vi "Get Spectrum.vi"(8 "error in (no error)":errorcluster, 11 "Micron Hyperion Driver in":refnum<class "Micron Hyperion Driver.lvclass">) -> (0 "error out":errorcluster, 2 "Spectrum Graph":cluster{dbl[], "Spectrum, db":dbl[]}[](graph), 3 "Micron Hyperion Driver out":refnum<class "Micron Hyperion Driver.lvclass">)   [LabVIEW 2016, in "Micron Hyperion Driver.lvclass"]
uses:
  Micron Hyperion Driver.lvclass
  Micron Hyperion Driver.lvclass/Micron Hyperion Driver.ctl
  Read Address.vi
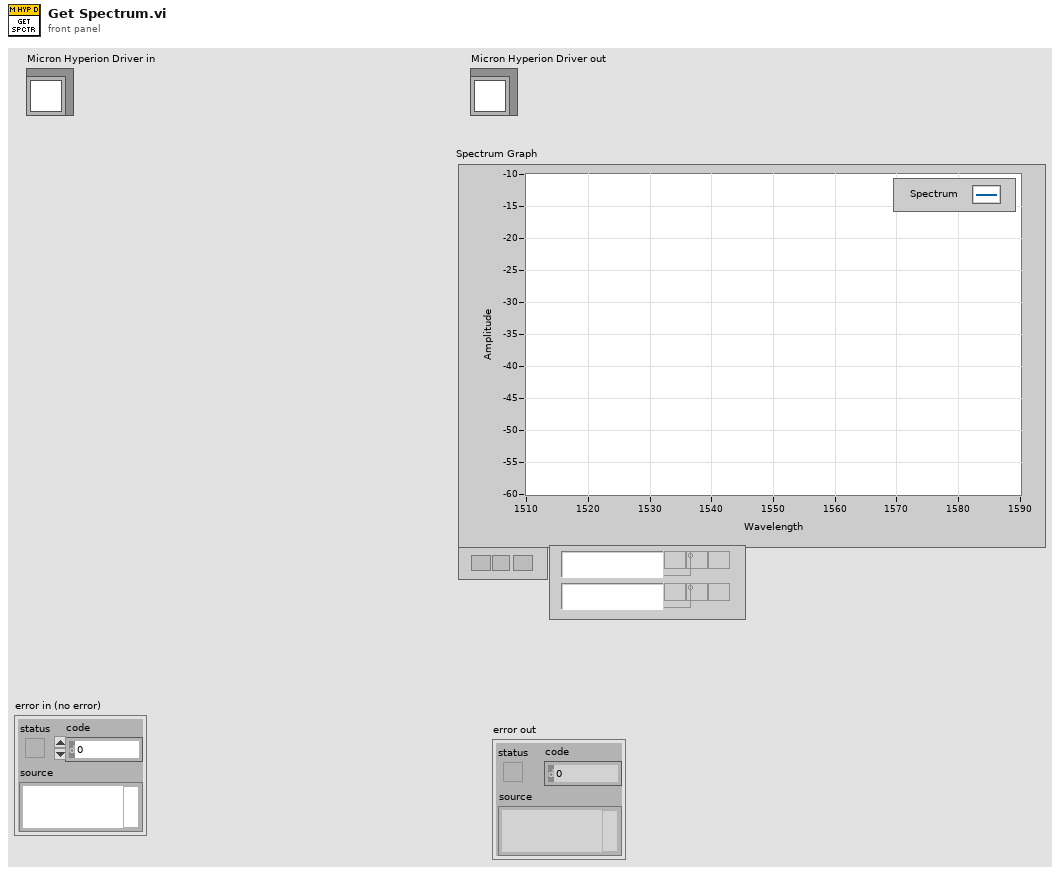
[diagram p1: front panel]
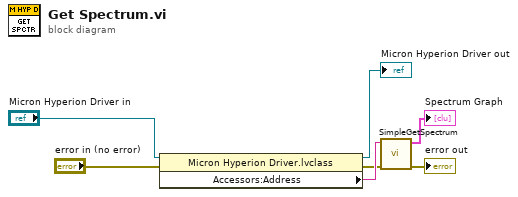
[diagram p0: block diagram]
diagram:
  n1 = property class="Micron Hyperion Driver.lvclass"(reference="Micron Hyperion Driver in", error in="error in (no error)") -> (reference out=→"Micron Hyperion Driver out":refnum<class "Micron Hyperion Driver.lvclass">, error out=w3:errorcluster, "Accessors:Address"=w4:string)
  n2 = call "SimpleGetSpectrum.vi"("Error In"=w3, "Address"=w4) -> ("Error Out"=→"error out":errorcluster, "Spectrum Graph"=→"Spectrum Graph":cluster{dbl[], "Spectrum, db":dbl[]}[])  [unwired: 6 in, 2 out]
